vi "update pixel clock slider.vi"(8 "error in (no error)":errorcluster, 11 "Thorcam in":refnum<class "Thorcam.lvclass">) -> (0 "error out":errorcluster, 3 "Thorcam out":refnum<class "Thorcam.lvclass">)   [LabVIEW 2012, in "Thorcam.lvclass"]
uses:
  Thorcam.lvclass
  Thorcam.lvclass/Thorcam.ctl
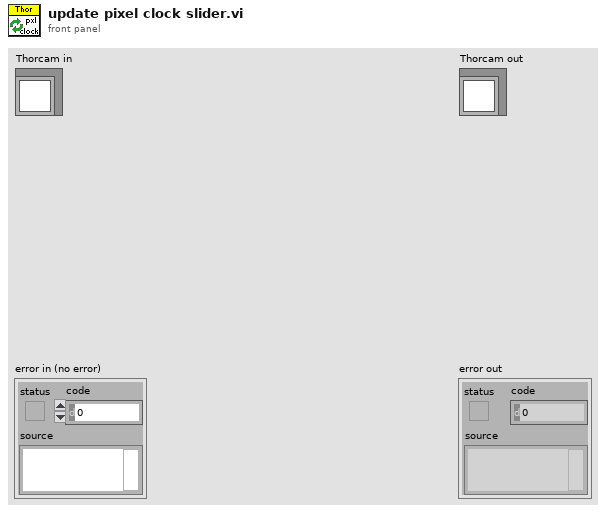
[diagram p1: front panel]
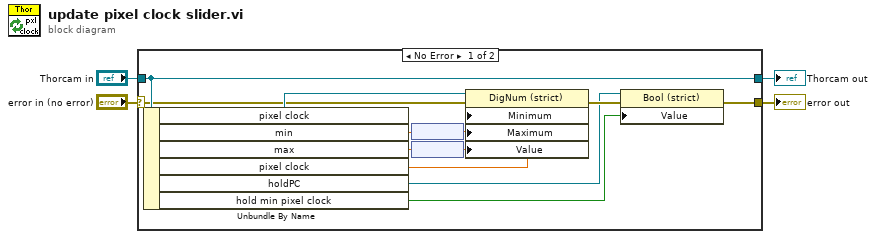
[diagram p0: block diagram]
diagram:
  n1 = case shown="No Error" "error in (no error)" {
    selector: "error in (no error)" -> [w14 w18]
    tunnel: [w7 w18] -> w3
    tunnel: [w15 w17] -> w1
    tunnel: "Thorcam in" -> [w15 w17]
    frame No Error {
      n2 = Unbundle By Name(w15) -> ("pixel clock"=w16:refnum<vi>, "min"=w12:dbl[unit], "max"=w11:dbl[unit], "pixel clock"=w13:dbl[unit], "holdPC"=w6:refnum<vi>, "hold min pixel clock"=w5:bool)
      n3 = node(w12) -> (w10:dbl)
      n4 = node(w11) -> (w9:dbl)
      n5 = property class="DigNum (strict)"(reference=w16, error in=w14, "Minimum"=w10, "Maximum"=w9, "Value"=w13) -> (error out=w8:errorcluster)  [unwired: 1 out]
      n6 = property class="Bool (strict)"(reference=w6, error in=w8, "Value"=w5) -> (error out=w7:errorcluster)  [unwired: 1 out]
    }
    frame Error {
    }
  }
  "error out" <- w3
  "Thorcam out" <- w1
